vi "Construct Event Source Filter.vi"(11 "Levels to Include (All)":T1={"Debug"=TRUE, "Info"=TRUE, "Warning"=TRUE, "Error"=TRUE, "Critical"=TRUE}) -> (3 "Event Level Filter out":refnum<class "Event Level Filter.lvclass">)   [LabVIEW 2020, in "Event Level Filter.lvclass"]
uses:
  <vilib>/gpm_packages/@cs/event-logger/Source/Filters/Event Level Filter/Event Level Filter.lvclass
  <vilib>/gpm_packages/@cs/event-logger/Source/Composed Log/Types/Log Level.ctl
  <vilib>/gpm_packages/@cs/event-logger/Source/Filters/Event Level Filter/Event Level Filter.lvclass/Event Level Filter.ctl
  <vilib>/gpm_packages/@cs/event-logger/Source/Composed Log/Composed Log.lvlib
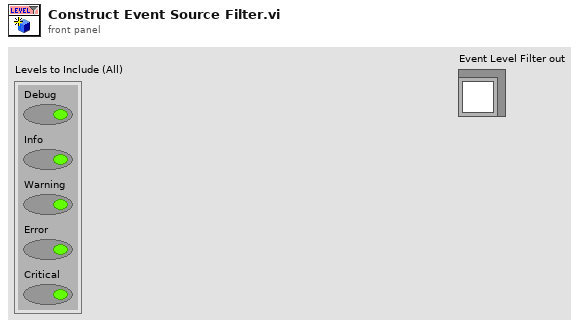
[diagram p1: front panel]
types:
  T1 = cluster{"Debug":bool, "Info":bool, "Warning":bool, "Error":bool, "Critical":bool}
  T2 = typedef "Composed Log.lvlib/Log Level.ctl" = enum16{"Debug", "Info", "Warning", "Error", "Critical"}
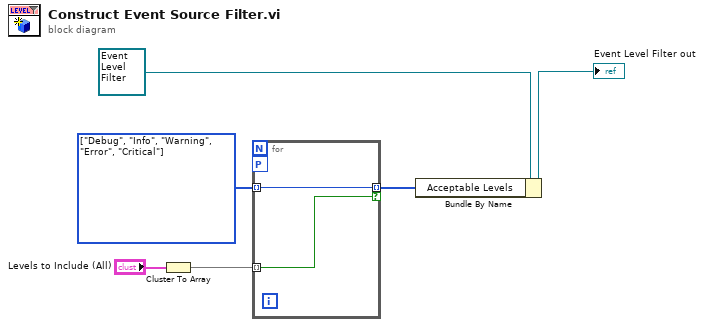
[diagram p0: block diagram]
diagram:
  w4 = T2[] [enum."Debug", enum."Info", enum."Warning", enum."Error", enum."Critical"] items=["Debug", "Info", "Warning", "Error", "Critical"] ("Acceptable Levels")
  n1 = Cluster To Array(cluster="Levels to Include (All)") -> (array=w1:bool[])
  n2 = for {
    tunnel: w4 -> [w8] mode=indexing
    tunnel: [w8] -> w3 mode=indexing if=w7
    tunnel: w1 -> [w7] mode=indexing
    workers-P: _ -> [_]
  }
  n3 = Bundle By Name(cluster=refnum<class "Event Level Filter.lvclass"> refnum ("Compound Filter in"), "Acceptable Levels"=w3) -> (→"Event Level Filter out":refnum<class "Event Level Filter.lvclass">)
